vi "SLL DE Check DO Interconn lines.vi"(6 "DO Interconnected lines":T1[][](array[typedef]), 9 "DO State Array In":bool[](array[boolean]), 10 "DO State":bool, 11 "DO Channel Name":T1) -> (1 "DO State Arra Out":bool[](array[boolean]))   [LabVIEW 2013]
uses:
  Controls/SLL DE List of Digital Outputs.ctl
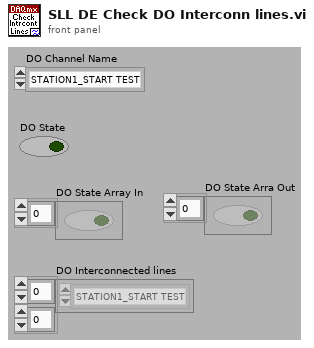
[diagram p1: front panel]
types:
  T1 = typedef "SLL DE List of Digital Outputs.ctl" = enum16{"STATION1_START TEST", "STATION1_STOP TEST", "STATION1_LIGHT1", "STATION1_LIGHT2", "STATION1_LIGHT3", "STATION1_SELECT_TEST", "STATION2_START TEST", "STATION2_STOP TEST", "STATION2_LIGHT1", "STATION2_LIGHT2", "STATION2_LIGHT3", "STATION2_SELECT_TEST", "STATION3_START TEST", "STATION3_STOP TEST", "STATION3_LIGHT1", "STATION3_LIGHT2", "STATION3_LIGHT3", "STATION3_SELECT_TEST", "STATION4_START TEST", "STATION4_STOP TEST", "STATION4_LIGHT1", "STATION4_LIGHT2", "STATION4_LIGHT3", "STATION4_SELECT_TEST"}
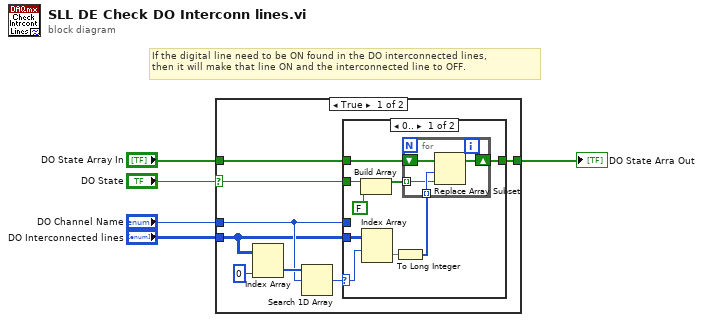
[diagram p0: block diagram]
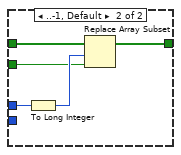
[diagram p2: hidden frame]
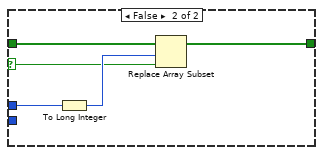
[diagram p3: hidden frame]
diagram:
  # "If the digital line need to be ON found in the DO interconnected lines,\nthen it will make that line ON and the interconnected line to OFF."
  n1 = case shown="True" "DO State" {
    selector: "DO State" -> [w10 w32]
    tunnel: [w13 w36] -> w1
    tunnel: "DO State Array In" -> [w12 w35]
    tunnel: "DO Channel Name" -> [w8 w34]
    tunnel: "DO Interconnected lines" -> [w6 _]
    frame True {
      n2 = Index Array(array=w6, index (col)=0 ("disabled index (col)")) -> (element=w9:T1[])  [unwired: 1 in]
      n3 = Search 1D Array(1D array=w9, element=w8) -> (index of element=w7:i32)  [unwired: 1 in]
      n4 = case shown="0.." w7 {
        selector: w7 -> [w21 _]
        tunnel: [w18 w31] -> w13
        tunnel: w12 -> [w19 w30]
        tunnel: w10 -> [w16 w28]
        tunnel: w8 -> [_ w27]
        tunnel: w6 -> [w22 _]
        frame 0.. {
          n5 = Build Array(w16, FALSE ("element")) -> (w15:bool[])
          n6 = Index Array(array=w22, index (row)=w21) -> (element=w20:T1[])  [unwired: 1 in]
          n7 = To Long Integer(number=w20) -> (32bit integer=w17:i32[])
          n8 = for {
            shift-right: [w25] -> w18
            shift-left: w19 -> [w26]
            tunnel: w17 -> [w24] mode=indexing
            tunnel: w15 -> [w23] mode=indexing
            n9 = Replace Array Subset(array=w26, new element=w23, index=w24) -> (w25:bool[])
          }
        }
        frame ..-1, Default {
          n10 = To Long Integer(number=w27) -> (32bit integer=w29:i32)
          n11 = Replace Array Subset(array=w30, new element=w28, index=w29) -> (w31:bool[])
        }
      }
    }
    frame False {
      n12 = To Long Integer(number=w34) -> (32bit integer=w33:i32)
      n13 = Replace Array Subset(array=w35, new element=w32, index=w33) -> (w36:bool[])
    }
  }
  "DO State Arra Out" <- w1
